vi "Read Test status.vi"(8 "error in (no error)":errorcluster, 11 "Fiber Auto Collimation state data in":refnum<class "Fiber Auto Collimation state data.lvclass">) -> (0 "error out":errorcluster, 2 "Test status":string, 3 "Fiber Auto Collimation state data out":refnum<class "Fiber Auto Collimation state data.lvclass">)   [LabVIEW 2018, in "Fiber Auto Collimation state data.lvclass"]
doc: "Gets the \"Test status\" string. Basically, a very short description of what's happening to keep the user informed."
uses:
  Fiber Auto Collimation state data.lvclass
  Fiber Auto Collimation state data.lvclass/Fiber Auto Collimation state data.ctl
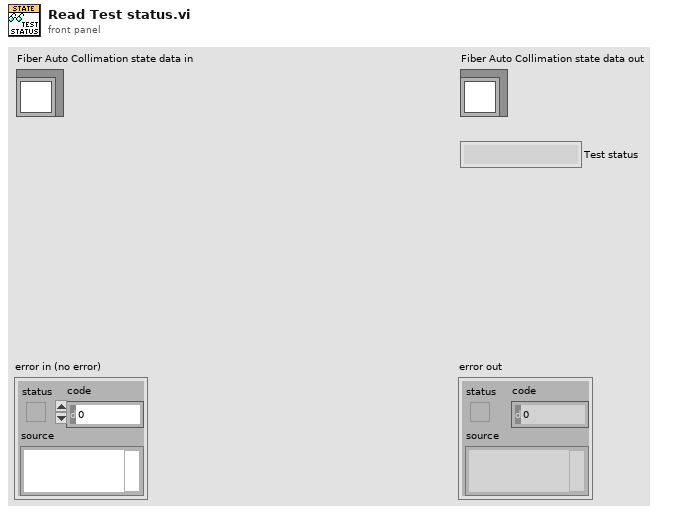
[diagram p1: front panel]
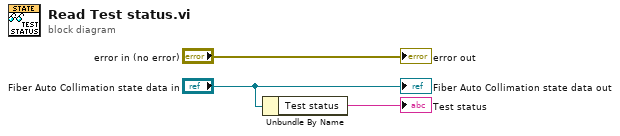
[diagram p0: block diagram]
diagram:
  n1 = Unbundle By Name("Fiber Auto Collimation state data in") -> ("Test status"=→"Test status":string)
  "error out" <- "error in (no error)"
  "Fiber Auto Collimation state data out" <- "Fiber Auto Collimation state data in"
